vi "DSF.Engine.Plugin.Obtain Transceiver Thread.vi"(8 "error in (no error)":errorcluster, 11 "Plugin in":refnum<class "DSF.Engine.Plugin.lvclass">) -> (0 "error out":errorcluster, 2 "Transceiver Thread":refnum<class "DSF.Engine.Transceiver Thread.lvclass">, 3 "Plugin out":refnum<class "DSF.Engine.Plugin.lvclass">)   [LabVIEW 2017, in "DSF.Engine.lvlib" / "DSF.Engine.Plugin.lvclass"]
uses:
  DSF.Engine.Plugin.lvclass
  Transceiver/DSF.Engine.Transceiver Thread.lvclass
  DSF.Engine.Plugin.lvclass/DSF.Engine.Plugin.ctl
  Thread Pool/DSF.Engine.Pool.ID.lvclass
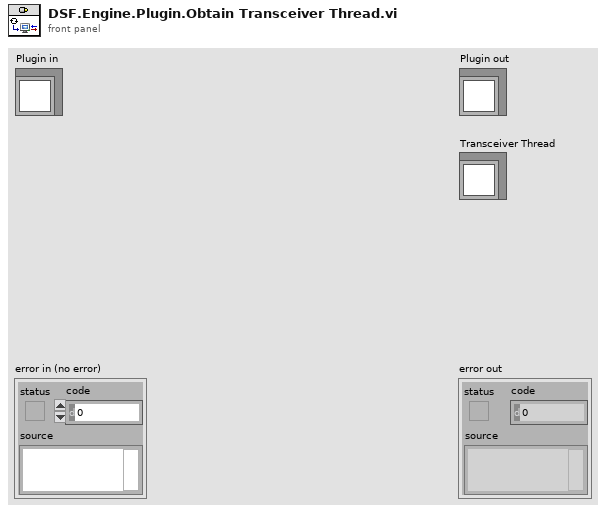
[diagram p1: front panel]
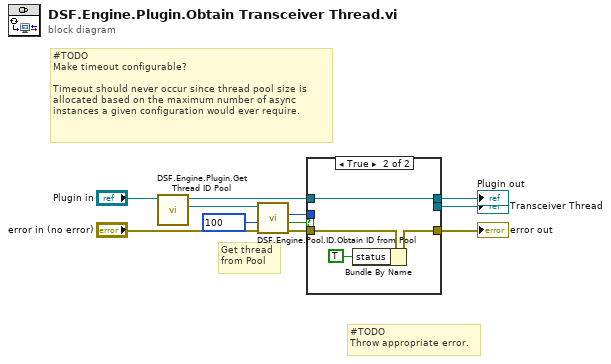
[diagram p0: block diagram]
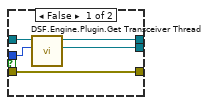
[diagram p2: hidden frame]
diagram:
  # "#TODO\nThrow appropriate error."
  # "#TODO\nMake timeout configurable?\n\nTimeout should never occur since thread pool size is allocated based on the maximum number of async instances a given configuration would ever require."
  # "Get thread from Pool"
  n1 = call "DSF.Engine.Plugin.Get Thread ID Pool.vi"("Plugin in"="Plugin in") -> ("Thread ID Pool"=w9:refnum<class "DSF.Engine.Pool.ID.lvclass">, "Plugin out"=w7:refnum<class "DSF.Engine.Plugin.lvclass">)  [unwired: 9 in]
  n2 = call "DSF.Engine.Pool.ID.Obtain ID from Pool.vi"("error in (no error)"="error in (no error)", "timeout in ms (0)"=100, "ID Pool in"=w9) -> ("error out"=w2:errorcluster, "timed out?"=w5:bool, "id"=w6:i32)  [unwired: 5 in, 1 out]
  n3 = case shown="True" w5 {
    tunnel: w7 -> [w16 w17]
    tunnel: w6 -> [w15 _]
    tunnel: [w14 w17] -> w4
    tunnel: [w13 _] -> w3
    tunnel: w2 -> [w12 w20]
    tunnel: [w12 w18] -> w1
    frame False {
      n4 = call "DSF.Engine.Plugin.Get Transceiver Thread.vi"("index"=w15, "Plugin in"=w16) -> ("Transceiver Thread"=w13:refnum<class "DSF.Engine.Transceiver Thread.lvclass">, "Plugin out"=w14:refnum<class "DSF.Engine.Plugin.lvclass">)  [unwired: 8 in]
    }
    frame True {
      n5 = Bundle By Name(cluster=w20, "status"=TRUE) -> (w18:errorcluster)
    }
  }
  "error out" <- w1
  "Plugin out" <- w4
  "Transceiver Thread" <- w3
